vi "WybierzPrzycisk.vi"(8 "error in":errorcluster, 11 "Wartość":T1) -> (0 "error out":errorcluster, 3 "Numer":u32)   [LabVIEW 2021]
doc: "Retrun the number of the button press"
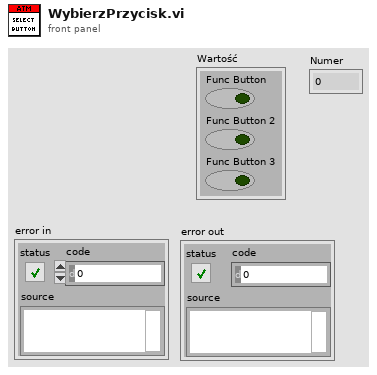
[diagram p1: front panel]
types:
  T1 = cluster{"Func Button":bool, "Func Button 2":bool, "Func Button 3":bool}
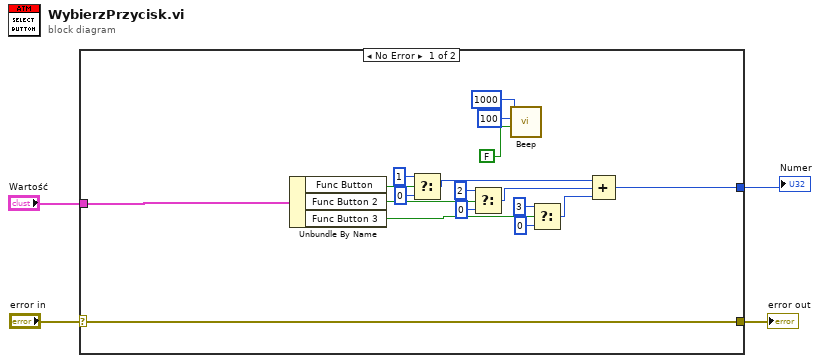
[diagram p0: block diagram]
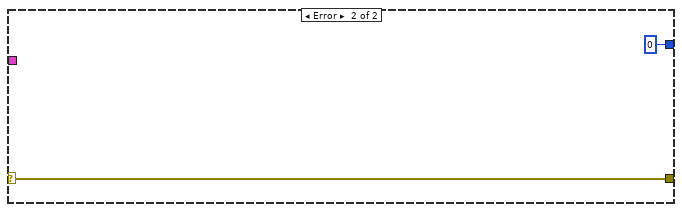
[diagram p2: hidden frame]
diagram:
  n1 = case shown="No Error" "error in" {
    selector: "error in" -> [w10 w23]
    tunnel: [w10 w23] -> w3
    tunnel: "Wartość" -> [w9 _]
    tunnel: [w8 u32 0] -> w1
    frame No Error {
      n2 = Unbundle By Name(w9) -> ("Func Button"=w11:bool, "Func Button 2"=w16:bool, "Func Button 3"=w19:bool)
      n3 = Select(t=u32 1, s=w11, f=u32 0) -> (s? t:f=w20:u32)
      n4 = Select(t=u32 2, s=w16, f=u32 0) -> (s? t:f=w21:u32)
      n5 = call <vilib>:"Beep.vi"("use system alert? (T)"=FALSE, "duration (msec)"=u32 100, "frequency (Hz)"=u32 1000) -> ()  [unwired: 9 in]
      n6 = Select(t=u32 3, s=w19, f=u32 0) -> (s? t:f=w22:u32)
      n7 = Compound Arithmetic op=ADD(w20, w21, w22) -> (w8:u32)
    }
    frame Error {
    }
  }
  "error out" <- w3
  "Numer" <- w1
